vi "Calculation average reflectance.vi"(9 "保存路径":path, 11 "file path (dialog if empty)":path) -> ()   [LabVIEW 2015]
uses:
  <vilib>/Utility/file.llb/Read Delimited Spreadsheet (string).vi
  <vilib>/Utility/file.llb/Write Delimited Spreadsheet (string).vi
panel:
  out "output array":string[][](array[string])
  out "all rows":string[][](array[string])
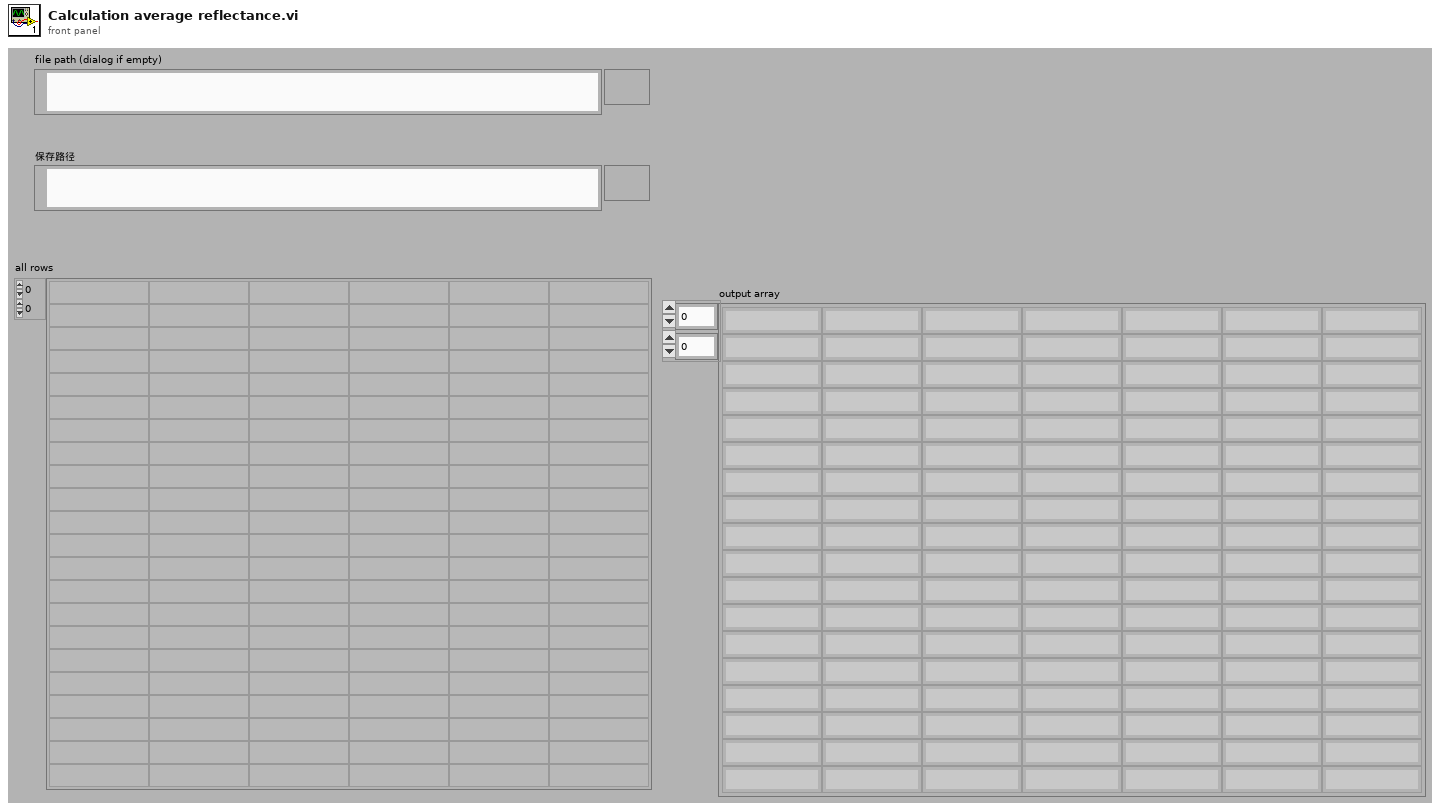
[diagram p1: front panel]
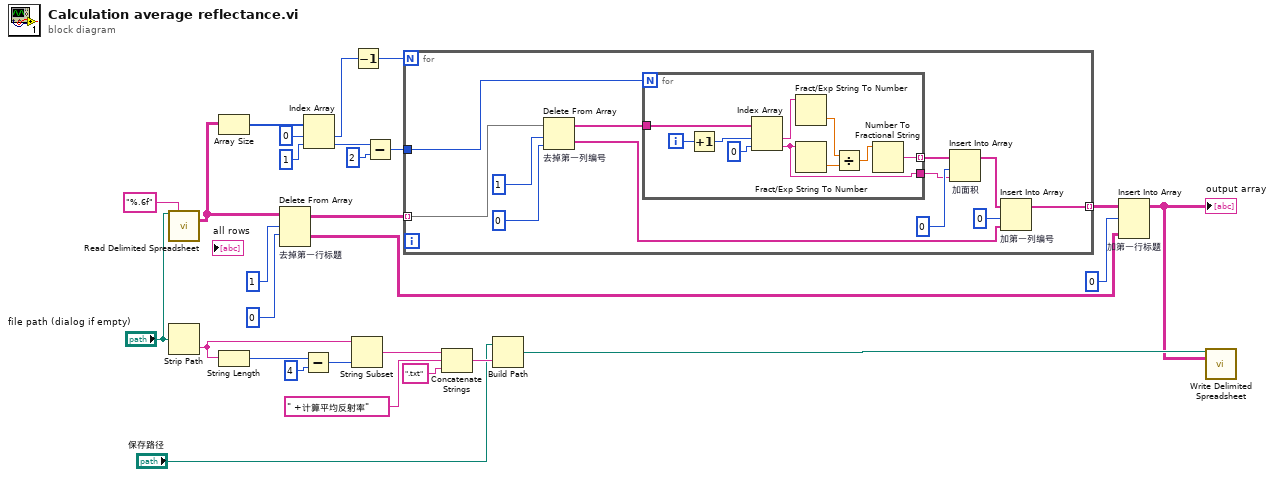
[diagram p0: block diagram]
diagram:
  n1 = call-poly <vilib>:"Read Delimited Spreadsheet.vi"("file path (dialog if empty)"="file path (dialog if empty)", "format (%s)"="%.6f" ("format (%.3f)")) -> ("all rows"=w3:string[][])  [unwired: 8 in, 5 out]
  n2 = Strip Path(path="file path (dialog if empty)") -> (name=w16:string)  [unwired: 1 out]
  n3 = Array Size(array=w3) -> (size(s)=w27:i32[])
  n4 = String Length(string=w16) -> (length=w15:i32)
  n5 = Delete From Array "去掉第一行标题"(array=w3, length=1, index (row)=0) -> (deleted portion=w18:string[][], array with subset deleted=w22:string[][])  [unwired: 1 in]
  n6 = Subtract(x=w15, y=4) -> (x-y=w13:i32)
  n7 = Index Array(array=w27, index #1=0 ("index"), index #2=1 ("index")) -> (element #1=w25:i32, element #2=w7:i32)
  n8 = String Subset(string=w16, length (rest)=w13) -> (substring=w10:string)  [unwired: 1 out]
  n9 = Decrement(x=w25) -> (x-1=w4:i32)
  n10 = Subtract(x=w7, y=2) -> (x-y=w5:i32)
  n11 = for {
    N: w4 -> [_]
    tunnel: w22 -> [w40] mode=indexing
    tunnel: w5 -> [w39]
    tunnel: [w31] -> w20 mode=indexing
    n12 = Delete From Array "去掉第一列编号"(array=w40, length=1, index=0) -> (deleted portion=w29:string[], array with subset deleted=w34:string[])
    n13 = for {
      N: w39 -> [_]
      tunnel: [w49] -> w38 mode=indexing
      tunnel: w34 -> [w48]
      tunnel: [w41] -> w33
      i -> [w47]
      n14 = Increment(x=w47) -> (x+1=w46:i32)
      n15 = Index Array(array=w48, index #1=w46, index #2=0 ("index")) -> (element #1=w44:string, element #2=w41:string)
      n16 = Fract/Exp String To Number(string=w44) -> (number=w43:dbl)  [unwired: 4 out]
      n17 = Fract/Exp String To Number(string=w41) -> (number=w42:dbl)  [unwired: 4 out]
      n18 = Divide(x=w43, y=w42) -> (x/y=w50:dbl)
      n19 = Number To Fractional String(number=w50) -> (F-format string=w49:string)  [unwired: 3 out]
    }
    n20 = Insert Into Array "加面积"(array=w38, index=0, new element=w33) -> (w32:string[])
    n21 = Insert Into Array "加第一列编号"(array=w32, index=0, new element=w29) -> (w31:string[])
  }
  n22 = Concatenate Strings(w10, " +计算平均反射率" ("string"), ".txt" ("string")) -> (w11:string)
  n23 = Build Path(base path="保存路径", name or relative path=w11) -> (appended path=w8:path)
  n24 = Insert Into Array "加第一行标题"(array=w20, index (row)=0, new element=w18) -> (w2:string[][])  [unwired: 1 in]
  "output array" <- w2
  n25 = call-poly <vilib>:"Write Delimited Spreadsheet.vi"("file path (dialog if empty)"=w8, "2D data"=w2) -> ()  [unwired: 12 in, 2 out]
